vi "validate.vi"(8 "error in":errorcluster, 11 "Thermo configuration in":refnum<class "Thermo configuration.lvclass">) -> (0 "error out":errorcluster, 3 "Thermo configuration out":refnum<class "Thermo configuration.lvclass">)   [LabVIEW 2025, in "Thermo.lvlib" / "Thermo configuration.lvclass"]
doc: "Provides an interface for performing validation on a given configuration. Any children should define the behavior of this function to ensure that the configuration in memory can be used by the runtime class.Copyright 2017 National Instruments Corporation\n\nLicensed under the Apache License, Version 2.0 (the \"License\"); you may not use this file except in compliance with the License. You may obtain a copy of the License at http://www.apache.org/licenses/LICENSE-2.0\nUnless required by applicable law or agreed to in writing, software distributed under the License is distributed on an \"AS IS\" BASIS, WITHOUT WARRANTIES OR CONDITIONS OF ANY KIND, either express or implied. See the License for the specific language governing permissions and limitations under the License."
uses:
  Thermo configuration.lvclass
  Users/Public/Documents/Sandia National Labs/TSS Plugin/Abstract Engine.lvlibp/Plugin/Abstract/Instrument configuration/Read Instrument Setting.vi
  Thermo configuration.lvclass/Thermo configuration.ctl
  Users/Public/Documents/Sandia National Labs/TSS Plugin/CEF.lvlibp
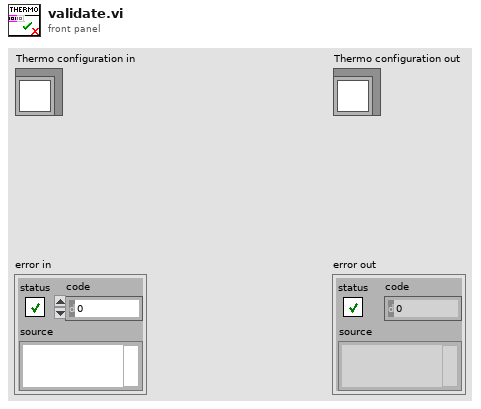
[diagram p1: front panel]
types:
  T1 = cluster{"Type":string, "Engine IP Address":string, "Engine Port":u32, "Address":string, "SW Alias":string, "Description":string, "Enabled":bool, "Model":string, "Serial Number":string, "Asset Number":string, "Calibration Date":string}
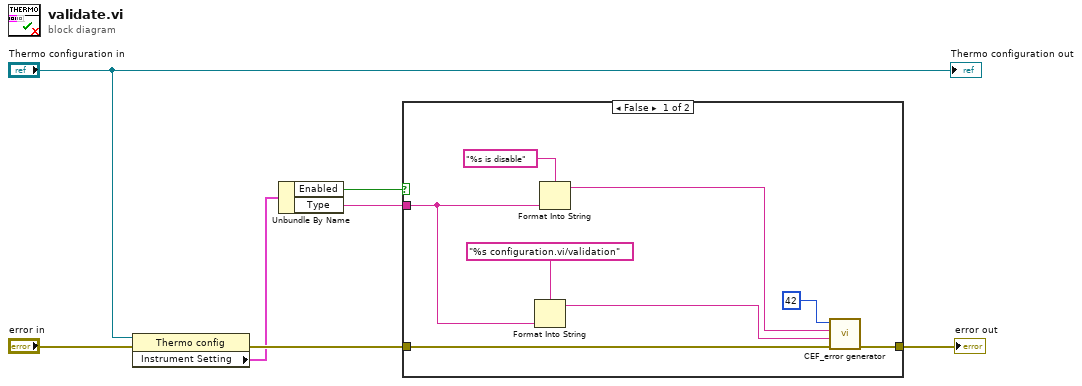
[diagram p0: block diagram]
diagram:
  n1 = property class="Thermo config"(reference="Thermo configuration in", error in="error in") -> (error out=w5:errorcluster, "Instrument Setting"=w3:T1)  [unwired: 1 out]
  n2 = Unbundle By Name(w3) -> ("Enabled"=w2:bool, "Type"=w1:string)
  n3 = case shown="False" w2 {
    tunnel: w5 -> [w15 w16]
    tunnel: [w14 w16] -> w6
    tunnel: w1 -> [w10 _]
    frame False {
      n4 = Format Into String(format string="%s configuration.vi/validation" ("source"), w10) -> (resulting string=w8:string)  [unwired: 2 in, 1 out]
      n5 = Format Into String(format string="%s is disable" ("append error message"), w10) -> (resulting string=w11:string)  [unwired: 2 in, 1 out]
      n6 = call "CEF_error generator.vi"("error in"=w15, "source"=w8, "append error message"=w11, "error code (0)"=42) -> ("error out"=w14:errorcluster)  [unwired: 5 in]
    }
    frame True {
    }
  }
  "error out" <- w6
  "Thermo configuration out" <- "Thermo configuration in"
